vi "Get All Component Settings.vi"(8 "error in (no error)":errorcluster, 11 "Runtime Configuration in":refnum<class "Runtime Configuration.lvclass">) -> (0 "error out":errorcluster, 2 "component settings":T1[](array[typedef]), 3 "Runtime Configuration out":refnum<class "Runtime Configuration.lvclass">)   [LabVIEW 2017, in "DSF Core.lvlib" / "Runtime Configuration.lvclass"]
uses:
  Runtime Configuration.lvclass
  Typedefs/DSF Settings Info.ctl
  Typedefs/DSF Version Info.ctl
  Runtime Configuration.lvclass/Runtime Configuration.ctl
  DSF Core.lvlib
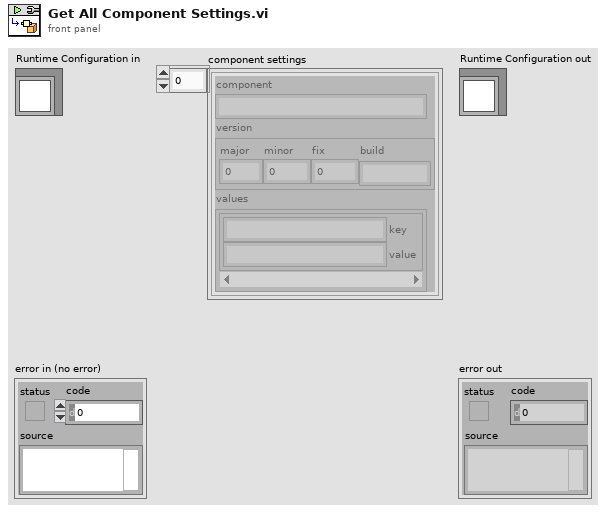
[diagram p1: front panel]
types:
  T1 = typedef "DSF Core.lvlib/DSF Settings Info.ctl" = cluster{"component":string, "version":T2, "values":cluster{"key":string, "value":string}[]}
  T2 = typedef "DSF Core.lvlib/DSF Version Info.ctl" = cluster{"major":u32, "minor":u32, "fix":u32, "build":string}
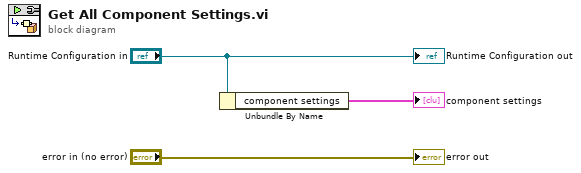
[diagram p0: block diagram]
diagram:
  n1 = Unbundle By Name("Runtime Configuration in") -> ("component settings"=→"component settings":T1[])
  "error out" <- "error in (no error)"
  "Runtime Configuration out" <- "Runtime Configuration in"
